vi "[Property] Cursors Write.vi"(4 "error in (no error)":errorcluster, 5 "Value":dbl[](array[numeric]), 6 "Container State":T2, 7 "Display State In":T1) -> (0 "error out":errorcluster, 3 "Display State Out":T1)   [LabVIEW 2014, in "Graph with cursors XControl.xctl"]
uses:
  Graph with cursors XControl.xctl
  <vilib>/_xctls/Container State.ctl
  Graph with cursors State.ctl
  <vilib>/_xctls/XControlSupport.lvlib
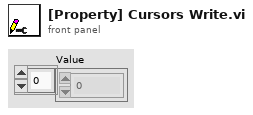
[diagram p1: front panel]
types:
  T1 = typedef "Graph with cursors XControl.xctl/Graph with cursors State.ctl" = cluster{"Cursor names":string[], "Cursor positions":dbl[], "Cursor pairs":i32, "Graph":refnum<vi>, "Prefix":string, "Base path":path}
  T2 = typedef "XControlSupport.lvlib/Container State.ctl" = cluster{"Indicator?":bool, "Run Mode?":bool, " Refnum":refnum<vi>}
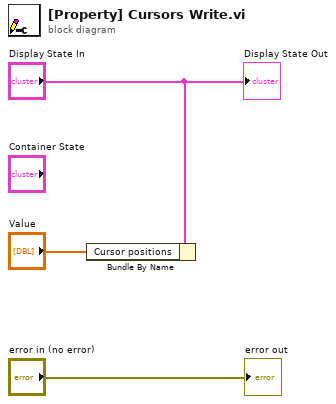
[diagram p0: block diagram]
diagram:
  n1 = Bundle By Name(cluster="Display State In", "Cursor positions"="Value") -> ()  [unwired: 1 out]
  "error out" <- "error in (no error)"
  "Display State Out" <- "Display State In"
